vi "Configure Carrier Component.vi"(5 "DMRS Type A Position (2)":i32=2, 6 "Physical Cell ID (0)":i32, 7 "Channel Bandwidth (50 MHz)":i32(ring) items=["50 MHz", "100 MHz", "200 MHz", "400 MHz"], 8 "error in (no error)":errorcluster, 9 "Carrier Component (1)":T1=1, 10 "Instance (1)":T2=1, 11 "VISA resource name":refnum<visa-resource-name>) -> (0 "error out":errorcluster, 3 "VISA resource name out":refnum<visa-resource-name>)   [LabVIEW 2015, in "Rohde&Schwarz CMXP NR FR2 Measurement.lvlib"]
doc: "Configures general parameters of carrier component.\n\nAttributes:\nRSCMXPNRFR2M_ATTR_CHANNEL_BANDWIDTH\nRSCMXPNRFR2M_ATTR_PHYSICAL_CELL_ID\nRSCMXPNRFR2M_ATTR_DMRS_TYPE_A_POSITION\n\nRemote-control commands:\nCONFigure:NRMMw:MEAS<i>[:CC<no>]:CBANdwidth\nCONFigure:NRMMw:MEAS<i>[:CC<no>]:PLCid\nCONFigure:NRMMw:MEAS<i>[:CC<no>]:TAPosition"
uses:
  <instrlib>/Rohde&Schwarz CMXP NR FR2 Measurement/Rohde&Schwarz CMXP NR FR2 Measurement.lvlib
  <instrlib>/Rohde&Schwarz CMXP NR FR2 Measurement/Private/_Instance.ctl
  <instrlib>/Rohde&Schwarz CMXP NR FR2 Measurement/Private/_Carrier Component.ctl
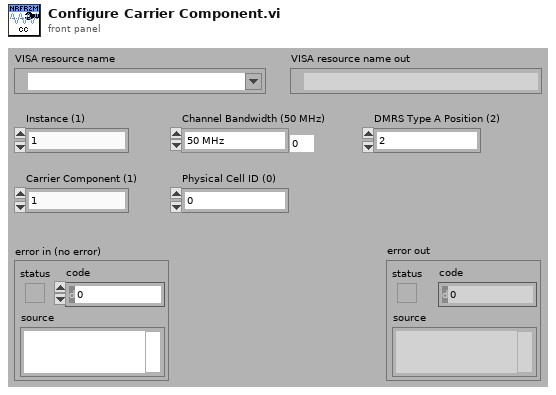
[diagram p1: front panel]
types:
  T1 = typedef "Rohde&Schwarz CMXP NR FR2 Measurement.lvlib/_Carrier Component.ctl" = i32
  T2 = typedef "Rohde&Schwarz CMXP NR FR2 Measurement.lvlib/_Instance.ctl" = i32
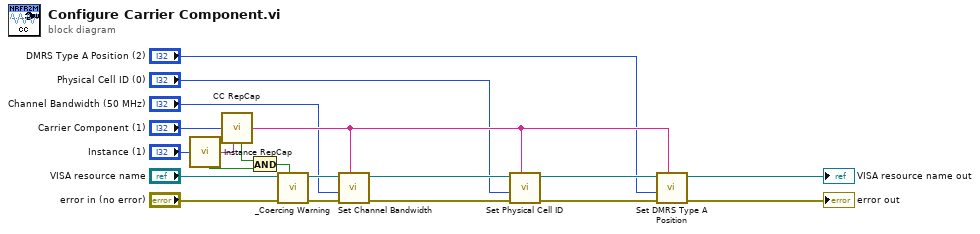
[diagram p0: block diagram]
diagram:
  n1 = call <instrlib>:"Instance RepCap.vi"("Instance In"="Instance (1)") -> ("In Range?"=w8:bool, "RepCap Identifier Out"=w4:string)  [unwired: 1 in]
  n2 = call <instrlib>:"CC RepCap.vi"("CC In"="Carrier Component (1)", "RepCap String In (\"\")"=w4) -> ("In Range?"=w9:bool, "RepCap Identifier Out"=w7:string)
  n3 = And(x=w9, y=w8) -> (x .and. y?=w12:bool)
  n4 = call <instrlib>:"_Coercing Warning.vi"("In Range?"=w12, "error in (no error)"="error in (no error)", "VISA resource name"="VISA resource name") -> ("error out"=w5:errorcluster, "VISA resource name out"=w6:refnum<visa-resource-name>)  [unwired: 7 in]
  n5 = call "Set Channel Bandwidth"("Repeated Capabilities"=w7, "error in (no error)"=w5, "Channel Bandwidth (0 - 50 MHz)"="Channel Bandwidth (50 MHz)", "instrument handle"=w6) -> ("error out"=w19:errorcluster, "instrument handle out"=w20:refnum<visa-resource-name>)  [unwired: 6 in]
  n6 = call "Set Physical Cell ID"("Repeated Capabilities"=w7, "error in (no error)"=w19, "Physical Cell ID (0)"="Physical Cell ID (0)", "instrument handle"=w20) -> ("error out"=w15:errorcluster, "instrument handle out"=w16:refnum<visa-resource-name>)  [unwired: 6 in]
  n7 = call "Set DMRS Type A Position"("Repeated Capabilities"=w7, "error in (no error)"=w15, "DMRS Type A Position (0)"="DMRS Type A Position (2)", "instrument handle"=w16) -> ("error out"=→"error out":errorcluster, "instrument handle out"=→"VISA resource name out":refnum<visa-resource-name>)  [unwired: 6 in]
